vi "Process.vi"(8 "error in":errorcluster, 11 "0MQ_Server":refnum<class "0MQ_Server.lvclass">) -> (0 "error out":errorcluster, 3 "0MQ_Server out":refnum<class "0MQ_Server.lvclass">)   [LabVIEW 2016, in "0MQ_Server.lvclass"]
doc: "---------------------------------------------------------------\nJKI State Machine Objects™\nhttp://jki.net/state-machine-objects/\nCopyright (C) 2005-2015, JKI <info@jki.net>\nALL RIGHTS RESERVED"
uses:
  0MQ_Server.lvclass
  C:/Program Files (x86)/National Instruments/LabVIEW 2016/vi.lib/JKI/JKI SMO/SMO/SMO.lvclass
  <vilib>/JKI/JKI SMO/SMO/Typedefs/Parent Call--Enum.ctl
  <vilib>/addons/zeromq/socket_type.ctl
  <vilib>/addons/zeromq/zmq_socket.lvclass
  <vilib>/addons/zeromq/zmq_context.lvclass
  0MQ_Server.lvclass/0MQ_Server.ctl
  <vilib>/addons/zeromq/socket_options.ctl
  <vilib>/JKI/JKI SMO/SMO/SMO.lvclass
  <vilib>/addons/zeromq/zeromq.lvlib
panel:
  # "For instructions on how to use the JKI State Machine Objects, examples and video tutorials, visit:\nhttp://jki.net/state-machine-objects/\n\nJKI State Machine Objects™\nhttp://jki.net/state-machine-objects/\nCopyright (C) 2005-2015, JKI <info@jki.net>\nALL RIGHTS RESERVED"
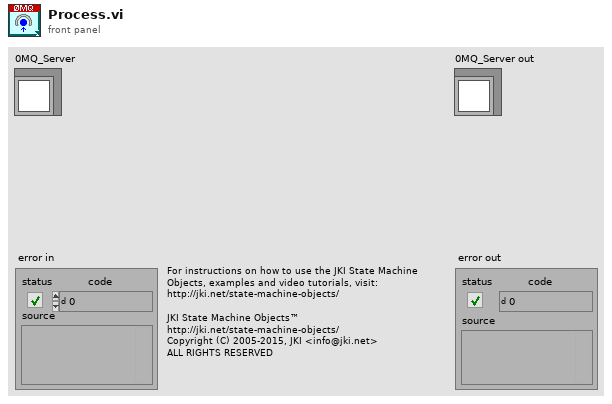
[diagram p1: front panel]
types:
  T1 = typedef "SMO.lvclass/Parent Call--Enum.ctl" = enum16{"Allows parent to run", "Does not request parent to run"}
  T2 = enum32{"invalid app kind", "Development System", "Run Time System", "Student Edition", "Embedded LabVIEW", "Evaluation", "Custom"}
  T3 = enum32{"Invalid", "Standard", "Closed", "Hidden", "Minimized", "Maximized"}
  T4 = enum32{"Bad", "Idle", "Run top level", "Running"}
  T5 = typedef "zeromq.lvlib/socket_options.ctl" = enum8{"NONE", "ZMQ_HWM", "<2>", "ZMQ_SWAP", "ZMQ_AFFINITY", "ZMQ_IDENTITY", "ZMQ_SUBSCRIBE", "ZMQ_UNSUBSCRIBE", "ZMQ_RATE", "ZMQ_RECOVERY_IVL", "ZMQ_MCAST_LOOP", "ZMQ_SNDBUF", "ZMQ_RCVBUF", "ZMQ_RCVMORE", "ZMQ_FD", "ZMQ_EVENTS", "ZMQ_TYPE", "ZMQ_LINGER", "ZMQ_RECONNECT_IVL", "ZMQ_BACKLOG", "ZMQ_RECOVERY_IVL_MSEC", "ZMQ_RECONNECT_IVL_MAX", "ZMQ_MAXMSGSIZE", "ZMQ_SNDHWM", "ZMQ_RCVHWM", "ZMQ_MULTICAST_HOPS", "<26>", "ZMQ_RCVTIMEO", "ZMQ_SNDTIMEO", "<29>", "<30>", "ZMQ_IPV4ONLY", "ZMQ_LAST_ENDPOINT", "ZMQ_ROUTER_MANDATORY", "ZMQ_TCP_KEEPALIVE", "ZMQ_TCP_KEEPALIVE_CNT", "ZMQ_TCP_KEEPALIVE_IDLE", "ZMQ_TCP_KEEPALIVE_INTVL", "ZMQ_TCP_ACCEPT_FILTER", "ZMQ_DELAY_ATTACH_ON_CONNECT", "ZMQ_XPUB_VERBOSE"}
  T6 = typedef "zeromq.lvlib/socket_type.ctl" = enum8{"ZMQ_PAIR", "ZMQ_PUB", "ZMQ_SUB", "ZMQ_REQ", "ZMQ_REP", "ZMQ_DEALER", "ZMQ_ROUTER", "ZMQ_PULL", "ZMQ_PUSH", "ZMQ_XPUB", "ZMQ_XSUB"}
  T7 = typedef "0MQ_Server.lvclass/Socket Config.ctl" = cluster{"Socket type":T6, "endpoint":string, "socket filter":string}
  T8 = cluster{"Core":cluster{"Current VI Reference":refnum<vi>, "Close Panel on Exit?":bool, "error":errorcluster}, "Self Reference":refnum<class "0MQ_Server.lvclass">, "ZMQ Socket":refnum<class "zmq_socket.lvclass">, "ZMQ Context":refnum<class "zmq_context.lvclass">, "Send String":string, "Socket Config":T7, "T_O":i32}
  T9 = cluster{"Current VI Reference":refnum<vi>, "Close Panel on Exit?":bool, "error":errorcluster}
  T10 = typedef "SMO.lvclass/Protected Events.ctl" = cluster{"StopProcesses":refnum<user-event>, "AbortProcesses":refnum<user-event>, "Config Changed":refnum<user-event>, "Dependency":refnum<user-event>}
  T11 = typedef "0MQ_Server.lvclass/0MQ_Server.ProtectedEvents.ctl" = cluster{"SendMessage":refnum<user-event>}
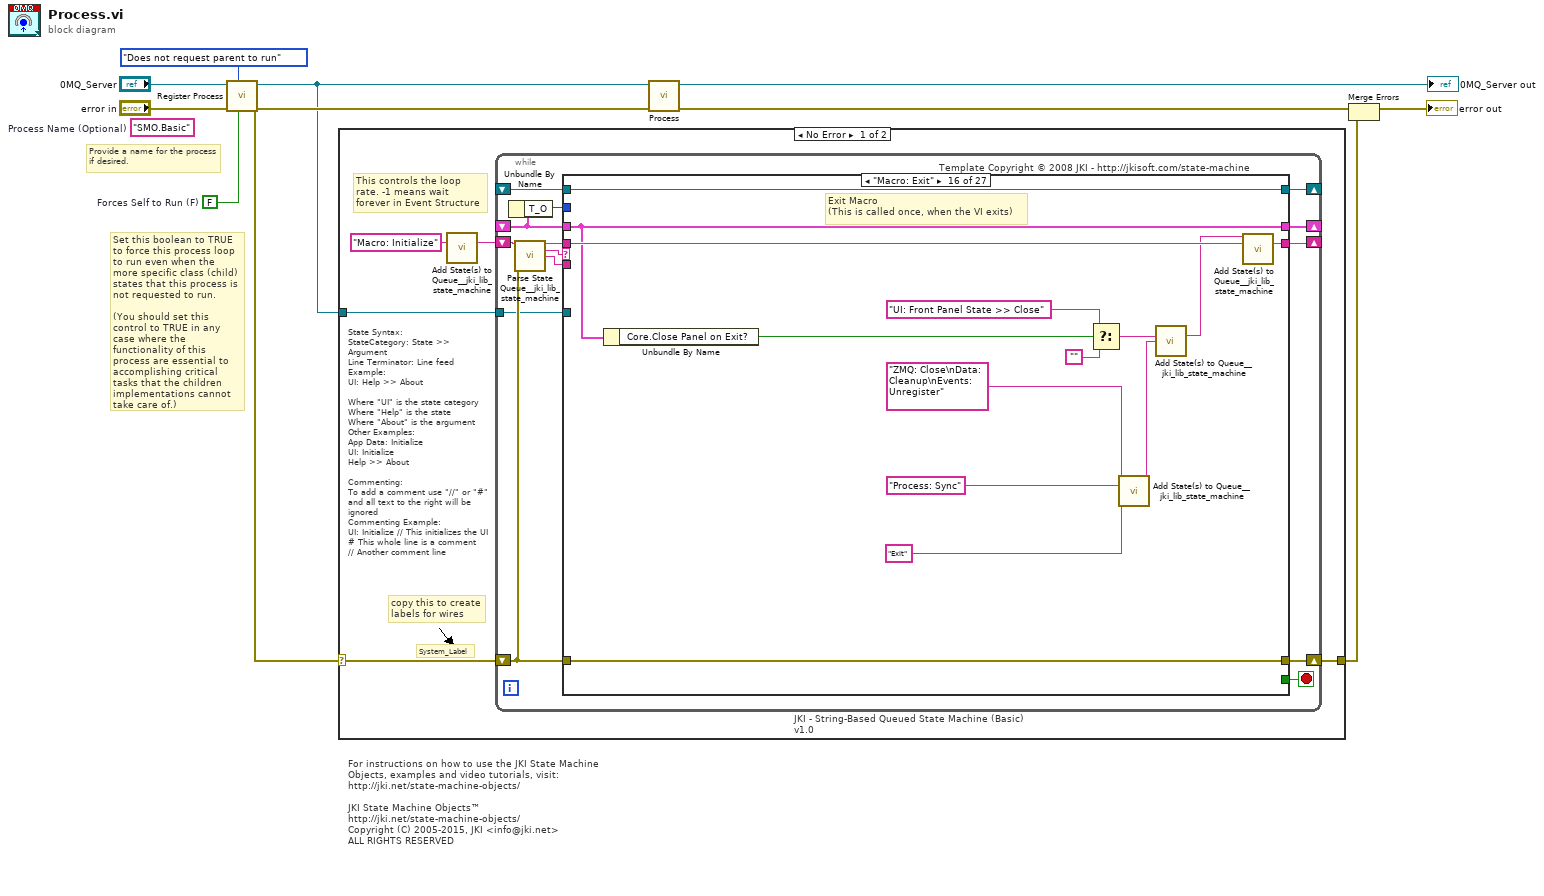
[diagram p0: block diagram]
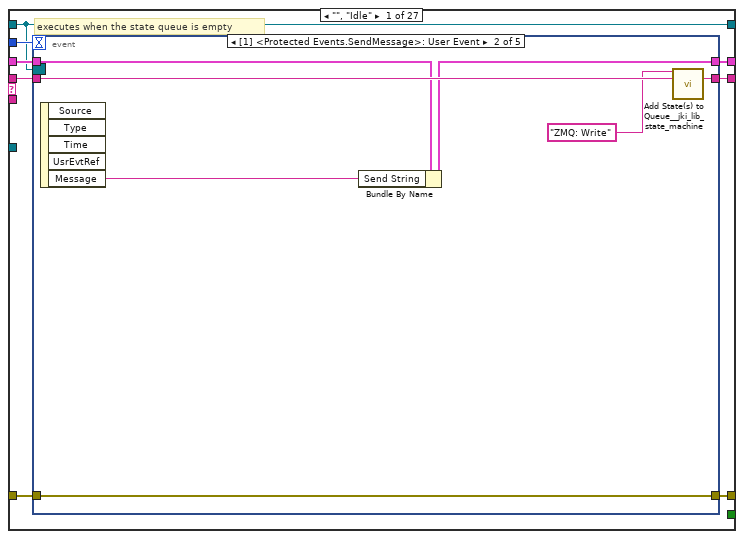
[diagram p2: hidden frame]
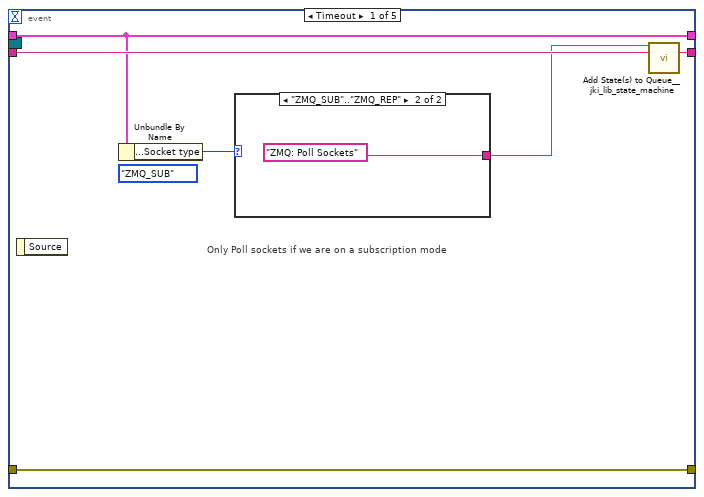
[diagram p3: hidden frame]
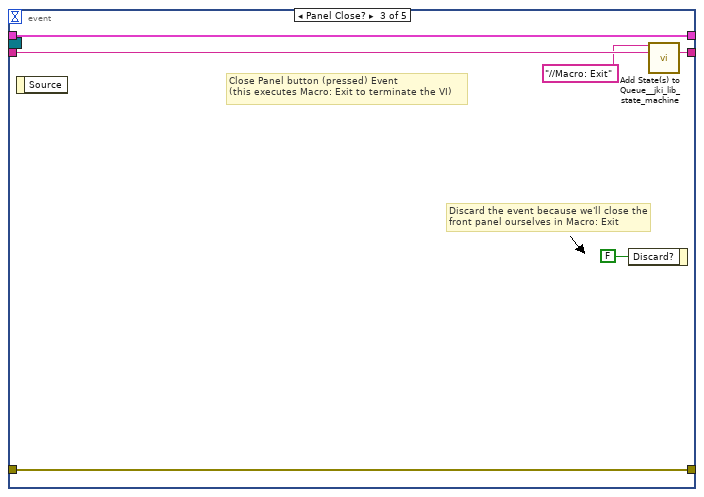
[diagram p5: hidden frame]
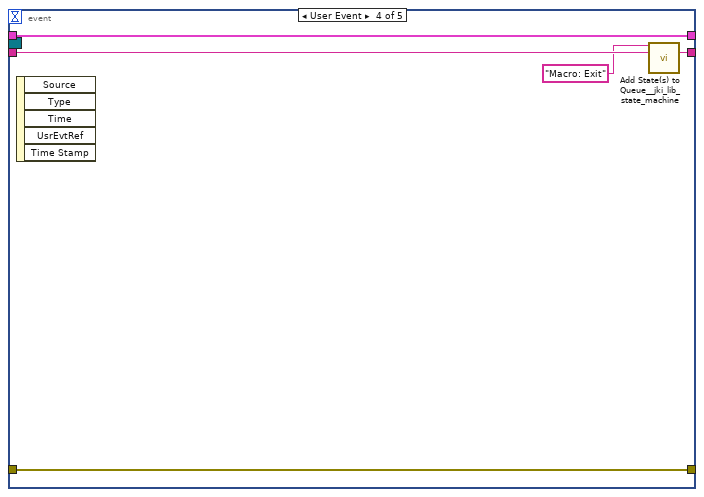
[diagram p6: hidden frame]
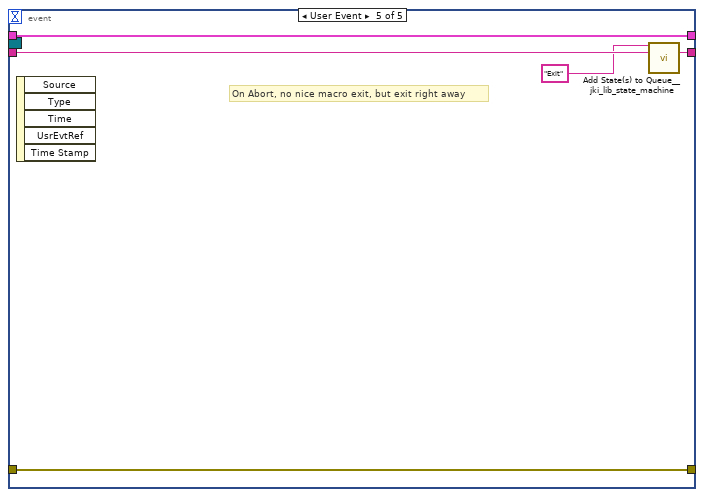
[diagram p7: hidden frame]
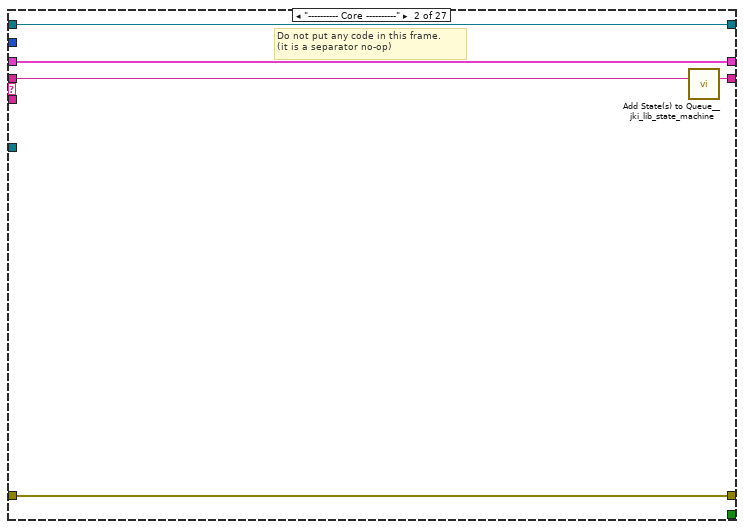
[diagram p8: hidden frame]
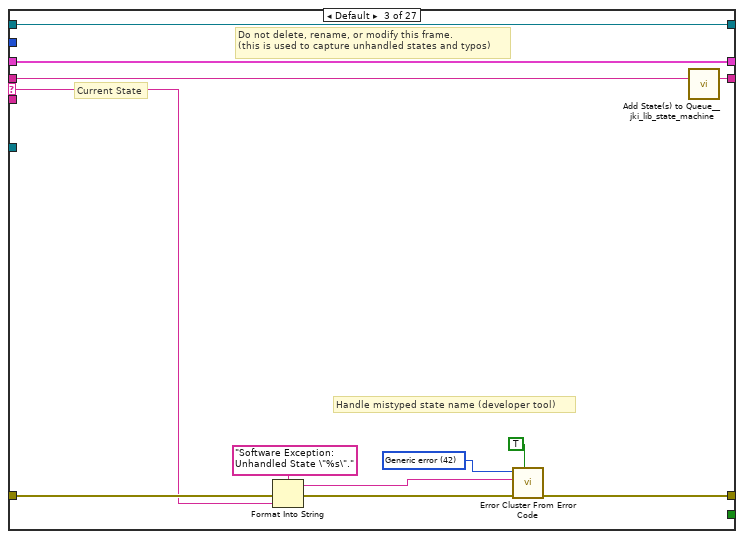
[diagram p9: hidden frame]
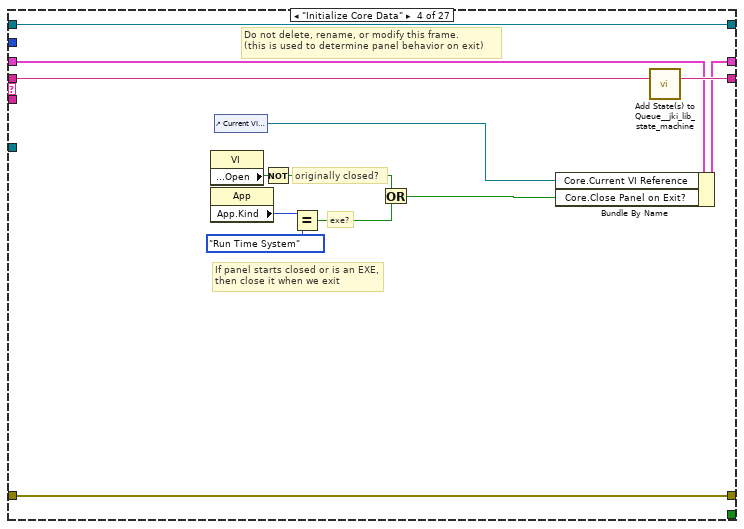
[diagram p10: hidden frame]
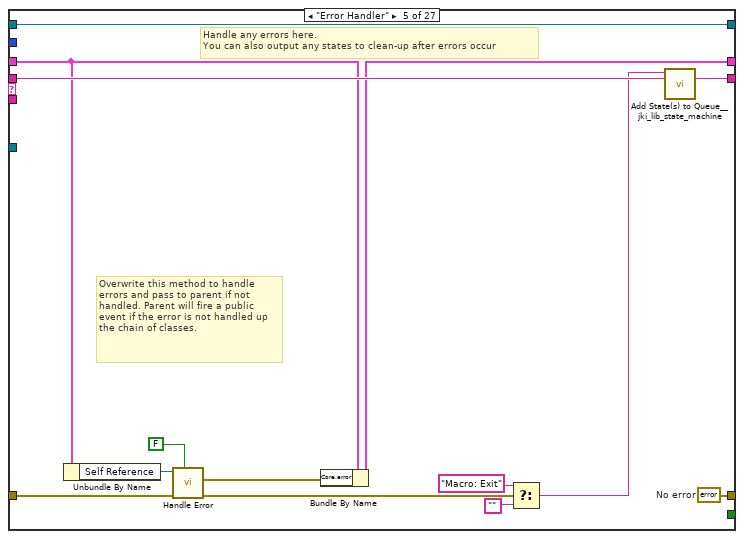
[diagram p11: hidden frame]
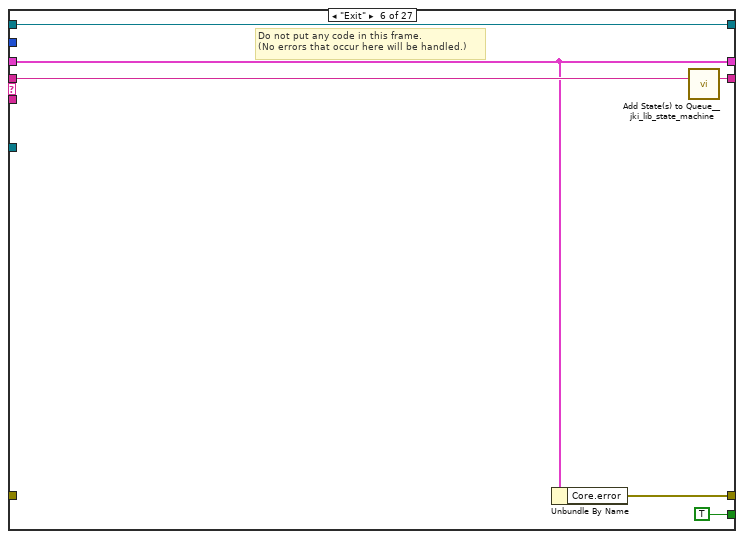
[diagram p12: hidden frame]
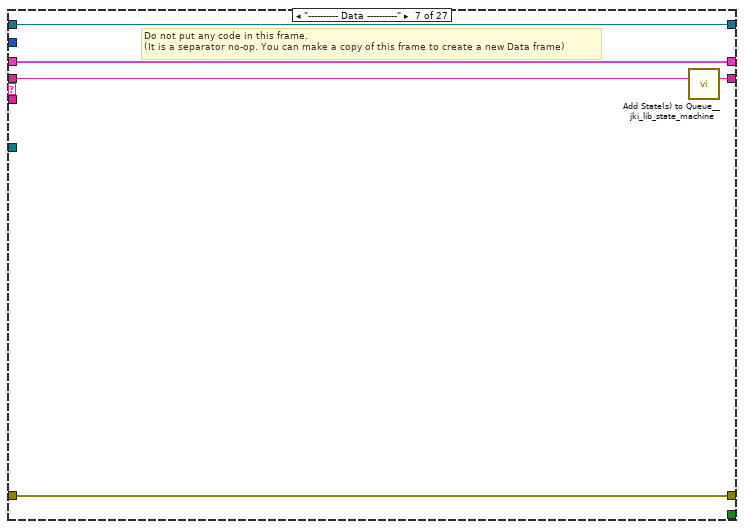
[diagram p13: hidden frame]
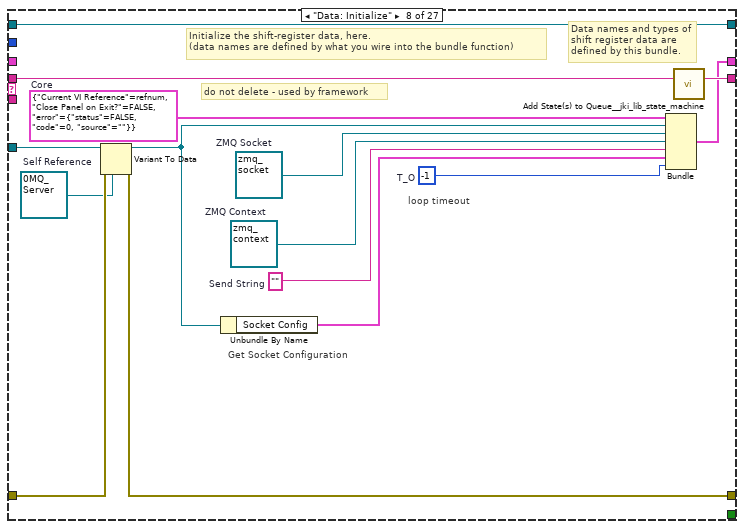
[diagram p14: hidden frame]
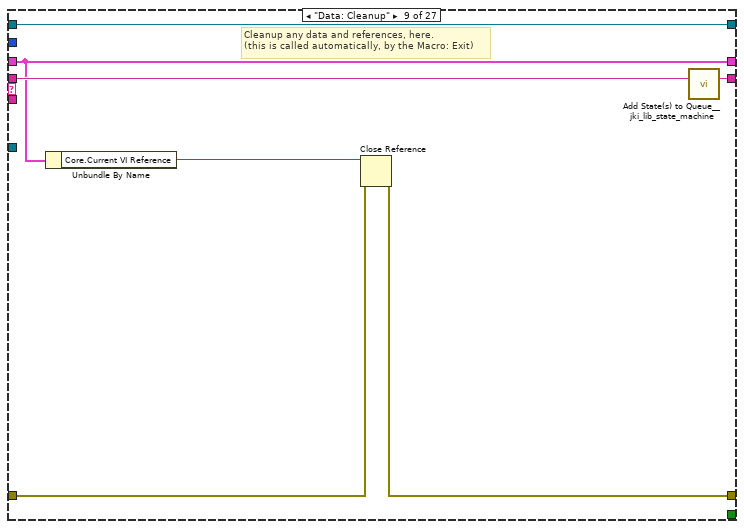
[diagram p15: hidden frame]
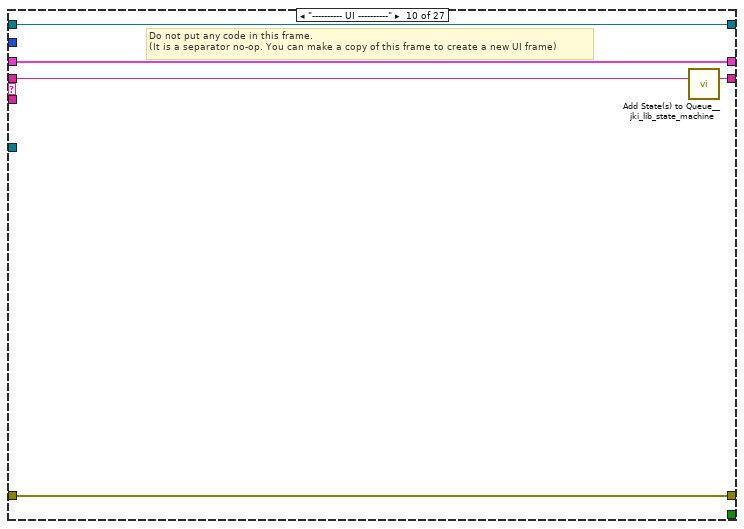
[diagram p16: hidden frame]
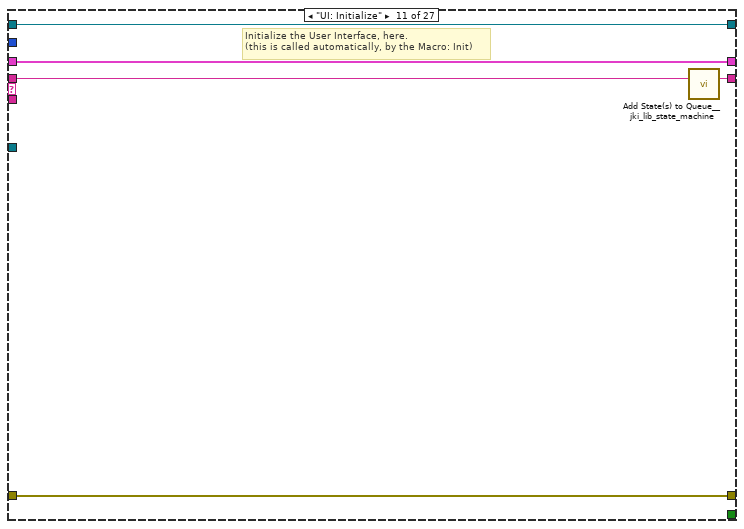
[diagram p17: hidden frame]
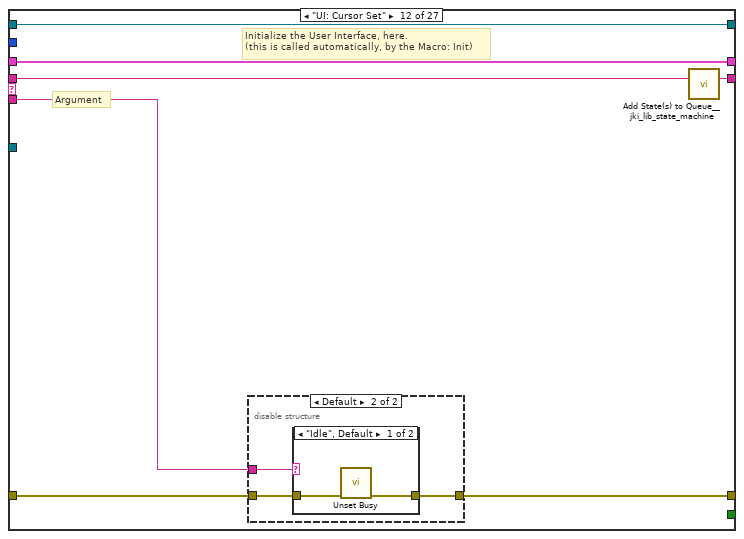
[diagram p18: hidden frame]
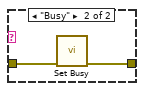
[diagram p20: hidden frame]
diagram:
  w1 = FALSE  # Forces Self to Run (F)
  (unwired) "SMO.Basic"  # Process Name (Optional)
  # "Provide a name for the process\nif desired."
  # "Set this boolean to TRUE to force this process loop to run even when the more specific class (child) states that this process is not requested to run.\n\n(You should set this control to TRUE in any case where the functionality of this process are essential to accomplishing critical tasks that the children implementations cannot take care of.)"
  # "For instructions on how to use the JKI State Machine Objects, examples and video tutorials, visit:\nhttp://jki.net/state-machine-objects/\n\nJKI State Machine Objects™\nhttp://jki.net/state-machine-objects/\nCopyright (C) 2005-2015, JKI <info@jki.net>\nALL RIGHTS RESERVED"
  n1 = call <vilib>:"Register Process.vi"("Forces Self to Run (F)"=w1, "Parent Call"=Parent_Call--Enum."Does not request parent to run", "error in (no error)"="error in", "SMO"="0MQ_Server") -> ("error out"=w7:errorcluster, "SMO out"=w6:refnum<class "0MQ_Server.lvclass">)  [unwired: 6 in]
  n2 = case shown="No Error" w7 {
    selector: w7 -> [w12 w391]
    tunnel: w6 -> [w13 _]
    tunnel: [w11 w391] -> w3
    frame No Error {
      # "State Syntax:\nStateCategory: State >> Argument\nLine Terminator: Line feed\nExample:\nUI: Help >> About\n\nWhere \"UI\" is the state category\nWhere \"Help\" is the state\nWhere \"About\" is the argument\nOther Examples:\nApp Data: Initialize\nUI: Initialize\nHelp >> About\n\nCommenting:\nTo add a comment use \"//\" or \"#\" and all text to the right will be ignored\nCommenting Example:\nUI: Initialize // This initializes the UI\n# This whole line is a comment\n// Another comment line"
      # "copy this to create labels for wires"
      # "This controls the loop rate. -1 means wait forever in Event Structure"
      # "System_Label"
      n3 = call <vilib>:"Add State(s) to Queue__jki_lib_state_machine.vi"("State(s) in (\"\")"="Macro: Initialize") -> ("States Out"=w15:string)  [unwired: 14 in]
      n4 = while "JKI - String-Based Queued State Machine (Basic) v1.0" {
        shift-right: [w22] -> _
        shift-left: _ -> [w17]
        shift-right: [w25] -> w11
        shift-left: w12 -> [w21]
        shift-right: [w24] -> _
        shift-left: w15 -> [w26]
        tunnel: w13 -> [w20]
        shift-right: [w19] -> _
        shift-left: _ -> [w18]
        stop <- w23 stop-if-true
        # "Template Copyright © 2008 JKI - http://jkisoft.com/state-machine"
        n5 = Unbundle By Name(w17) -> ("T_O"=w16:i32)
        n6 = call <vilib>:"Parse State Queue__jki_lib_state_machine.vi"("State Queue"=w26, "Error In (no error)"=w21) -> ("Remaining States"=w28:string, "Current State"=w29:string, "Arguments"=w27:string)  [unwired: 11 in]
        n7 = case shown="\"Macro: Exit\"" w29 {
          selector: w29 -> [_ _ w74 _ _ _ _ _ _ _ _ _ _ _ _ _ _ _ _ _ _ _ _ _ _ _ _]
          tunnel: w28 -> [w37 w72 w78 w97 w111 w117 w122 w137 w144 w149 w154 w161 w177 w209 w223 w237 w242 w253 w258 w272 w288 w293 w305 w318 w358 w367 w384]
          tunnel: w27 -> [_ _ _ _ _ _ _ _ _ _ _ w155 w171 _ _ _ _ _ _ _ _ _ _ _ _ _ _]
          tunnel: w17 -> [w35 w69 w76 w88 w100 w113 w119 _ w139 w146 w152 w159 w173 w206 w219 w228 w239 w250 w255 w270 w286 w291 w294 w314 w354 w364 w381]
          tunnel: [w34 w70 w80 w94 w102 w112 w120 w133 w140 w147 w151 w156 w174 w207 w221 w235 w240 w244 w256 w268 w283 w289 w296 w309 w351 w361 w379] -> w25
          tunnel: w21 -> [w33 w70 w79 w94 w107 _ w120 w134 w141 w147 w151 w157 w175 w207 w221 w235 w240 w245 w256 w269 w284 w289 w297 w310 w352 w362 w380]
          tunnel: [w36 w71 w77 w96 w110 w116 w121 w136 w143 w148 w153 w160 w176 w208 w222 w236 w241 w252 w257 w271 w287 w292 w304 w317 w357 w366 w383] -> w24
          tunnel: [_ _ _ _ _ TRUE _ _ _ _ _ _ _ _ _ _ _ _ _ _ _ _ _ _ _ _ _] -> w23
          tunnel: [w32 w69 w76 w95 w99 w113 w119 w135 w139 w146 w152 w159 w173 w206 w219 w228 w239 w250 w255 w270 w286 w291 w300 w315 w354 w364 w381] -> w22
          tunnel: w16 -> [w31 _ _ _ _ _ _ _ _ _ _ _ _ _ _ _ _ _ _ _ _ _ _ _ _ _ _]
          tunnel: w20 -> [_ _ _ _ _ _ _ w131 _ _ _ _ _ _ _ _ _ _ _ _ _ _ _ _ _ _ _]
          tunnel: [w30 w68 w73 w85 w109 w114 w118 w130 w138 w145 w150 w158 w170 w205 w220 w229 w238 w251 w254 w267 w285 w290 w303 w316 w356 w365 w382] -> w19
          tunnel: w18 -> [w30 w68 w73 w85 w109 w114 w118 w130 w138 w145 w150 w158 w170 w205 w220 w229 w238 w251 w254 w263 w285 w290 w303 w316 w356 w365 w382]
          frame "", "Idle" {
            # "executes when the state queue is empty"
            n8 = event shown="[1] <Protected Events.SendMessage>: User Event" {
              selector: w30 -> [_ _ _ _ _]
              dyn-events: _ -> [_ _ _ _ _]
              timeout: w31 -> [_ _ _ _ _]
              tunnel: w37 -> [w43 w51 w57 w62 w67]
              tunnel: [w42 w50 w56 w61 w66] -> w36
              tunnel: w35 -> [w40 w48 w54 w59 w64]
              tunnel: [w41 w49 w55 w60 w65] -> w34
              tunnel: w33 -> [w41 w49 w55 w60 w65]
              tunnel: [w40 w47 w54 w59 w64] -> w32
              event Timeout {
                (unwired) socket_type."ZMQ_SUB" ("y")
                # "Only Poll sockets if we are on a subscription mode"
                n9 = event-data() -> ()  [unwired: 1 in, 1 out]
                n10 = Unbundle By Name(w40) -> ("Socket Config.Socket type"=w38:T6)
                n11 = case shown="\"ZMQ_SUB\"..\"ZMQ_REP\"" w38 {
                  tunnel: [_ "ZMQ: Poll Sockets" ("State(s) in Front (\"\")")] -> w39
                  frame Default {
                  }
                  frame "ZMQ_SUB".."ZMQ_REP" {
                  }
                }
                n12 = call <vilib>:"Add State(s) to Queue__jki_lib_state_machine.vi"("State(s) in Front (\"\")"=w39, "State(s) in (\"\")"=w43) -> ("States Out"=w42:string)  [unwired: 13 in]
              }
              event User Event {
                n13 = event-data() -> ("Message"=w46:string)  [unwired: 1 in, 4 out]
                n14 = Bundle By Name(cluster=w48, "Send String"=w46) -> (w47:T8)
                n15 = call <vilib>:"Add State(s) to Queue__jki_lib_state_machine.vi"("State(s) in Front (\"\")"="ZMQ: Write" ("State(s) in Front (\"\")"), "State(s) in (\"\")"=w51) -> ("States Out"=w50:string)  [unwired: 13 in]
              }
              event Panel Close? {
                # "Discard the event because we'll close the front panel ourselves in Macro: Exit"
                # "Close Panel button (pressed) Event\n(this executes Macro: Exit to terminate the VI)"
                n16 = event-data() -> ()  [unwired: 1 in, 1 out]
                n17 = event-data("Discard?"=FALSE) -> ()  [unwired: 1 in, 1 out]
                n18 = call <vilib>:"Add State(s) to Queue__jki_lib_state_machine.vi"("State(s) in Front (\"\")"="//Macro: Exit", "State(s) in (\"\")"=w57) -> ("States Out"=w56:string)  [unwired: 13 in]
              }
              event User Event {
                n19 = event-data() -> ()  [unwired: 1 in, 5 out]
                n20 = call <vilib>:"Add State(s) to Queue__jki_lib_state_machine.vi"("State(s) in Front (\"\")"="Macro: Exit", "State(s) in (\"\")"=w62) -> ("States Out"=w61:string)  [unwired: 13 in]
              }
              event User Event {
                # "On Abort, no nice macro exit, but exit right away"
                n21 = event-data() -> ()  [unwired: 1 in, 5 out]
                n22 = call <vilib>:"Add State(s) to Queue__jki_lib_state_machine.vi"("State(s) in Front (\"\")"="Exit", "State(s) in (\"\")"=w67) -> ("States Out"=w66:string)  [unwired: 13 in]
              }
            }
          }
          frame "---------- Core ----------" {
            # "Do not put any code in this frame.\n(it is a separator no-op)"
            n23 = call <vilib>:"Add State(s) to Queue__jki_lib_state_machine.vi"("State(s) in (\"\")"=w72) -> ("States Out"=w71:string)  [unwired: 14 in]
          }
          frame Default {
            w83 = 42 items=["No error", "Argument error", "Memory is full", "Out of zone", "End of file", "File already open", "Generic file I/O error", "File not found", "File permission error", "Disk is full", "Duplicate path", "Too many files open", "System feature not enabled", "Resource file not found", "Cannot add resource", "Resource not found", "Image not found", "Image memory error", "Pen does not exist", "Config type invalid", "Config token not found", "Config parse error", "Config memory error", "Bad external code format", "Bad external code offset", "External code not present", "Null window", "Destroy window error", "Null menu", "Print aborted", "Bad print record", "Print driver error", "Windows error during printing", "Memory error during printing", "Print dialog error", "Generic print error", "Invalid device refnum", "Device not found", "Device parameter error", "Device unit error", "Cannot open device", "Device call aborted", "Generic error", "Cancelled by user", "Object ID too low", "Object ID too high", "Object not in heap", "Unknown heap", "Unknown object (invalid DefProc)", "Unknown object (DefProc not in table)", "Message out of range", "Invalid (null) method", "Unknown message", "Manager call not supported", "Bad address", "Network operation in progress", "Network operation timed out", "Connection is busy", "Network attribute not supported", "Network error", "Address in use", "System out of memory", "Connection aborted", "Connection refused", "Not connected", "Already connected", "Connection closed", "Initialization error (interapplication manager)", "Bad occurrence", "Wait on unbound occurrence handler", "Occurrence queue overflow", "Datalog type conflict", "Unused", "Unrecognized type (interapplication manager)", "Memory corrupt", "Failed to make temporary DLL", "Old CIN version", "Drag socket not found", "Failed to load drop-object", "Failed to register OLE object", "Failed to release OLE object", "Format specifier type mismatch", "Unknown format specifier", "Too few format specifiers", "Too many format specifiers", "Scan failed", "Newer CIN version", "Error converting to variant", "Runtime menu error", "Password tampered", "Variant attribute not found", "Incompatible variant data type", "Event data is not available", "Event Store is not present", "Occurrence is not found", "Event Queue is not created", "Event info is not available", "Refnum passed is NULL", "Error retrieving Class GUID", "Error retrieving CoClass GUID", "Error retrieving TypeLib GUID.", "Bad built application magic bytes.", "Specific driver is different from the specific driver associated with the Logical Name.", "There is no session opened to the class driver.", "Max Error", "MAX - Error with config objects", "MAX - Error loading configuration", "MAX - Group not supported"]
            # "Current State"
            # "Do not delete, rename, or modify this frame.\n(this is used to capture unhandled states and typos)"
            # "Handle mistyped state name (developer tool)"
            n24 = Format Into String(format string="Software Exception: Unhandled State \"%s\"." ("message"), error in=w79, w74) -> (resulting string=w82:string, error out=w81:errorcluster)  [unwired: 1 in]
            n25 = call <vilib>:"Error Cluster From Error Code.vi"("show call chain? (False)"=TRUE, "error in (no error)"=w81, "error message (\"\")"=w82, "error code (0)"=w83) -> ("error out"=w80:errorcluster)  [unwired: 5 in]
            n26 = call <vilib>:"Add State(s) to Queue__jki_lib_state_machine.vi"("State(s) in (\"\")"=w78) -> ("States Out"=w77:string)  [unwired: 14 in]
          }
          frame "Initialize Core Data" {
            # "Do not delete, rename, or modify this frame.\n(this is used to determine panel behavior on exit)"
            # "originally closed?"
            # "exe?"
            # "If panel starts closed or is an EXE, then close it when we exit"
            n27 = property class="VI"() -> ("Front Panel.Open"=w93:bool)  [unwired: 2 in, 2 out]
            n28 = property class="App"() -> ("App.Kind"=w92:T2)  [unwired: 2 in, 2 out]
            n29 = control-ref of="Current VI Reference"() -> (w86:refnum<vi>)
            n30 = Not(x=w93) -> (.not. x?=w90:bool)
            n31 = Equal?(x=w92, y=T2."Run Time System" ("Application:Kind")) -> (x = y?=w89:bool)
            n32 = Or(x=w90, y=w89) -> (x .or. y?=w87:bool)
            n33 = Bundle By Name(cluster=w88, "Core.Current VI Reference"=w86, "Core.Close Panel on Exit?"=w87) -> (w95:T8)
            n34 = call <vilib>:"Add State(s) to Queue__jki_lib_state_machine.vi"("State(s) in (\"\")"=w97) -> ("States Out"=w96:string)  [unwired: 14 in]
          }
          frame "Error Handler" {
            w102 = errorcluster {"status"=FALSE, "code"=0, "source"=""}  # No error
            # "Overwrite this method to handle errors and pass to parent if not handled. Parent will fire a public event if the error is not handled up the chain of classes."
            # "Handle any errors here.\nYou can also output any states to clean-up after errors occur"
            n35 = Unbundle By Name(w100) -> ("Self Reference"=w108:refnum<class "0MQ_Server.lvclass">)
            n36 = call-dynamic "Handle Error.vi"("Stop on Unhandled Error (T)"=FALSE, "error in"=w107, "SMO"=w108) -> ("handling error"=w103:errorcluster, "Unhandled error"=w101:errorcluster)  [unwired: 6 in, 1 out]
            n37 = Bundle By Name(cluster=w100, "Core.error"=w101) -> (w99:T8)
            n38 = Select(t="Macro: Exit", s=w103, f="") -> (s? t:f=w104:string)
            n39 = call <vilib>:"Add State(s) to Queue__jki_lib_state_machine.vi"("State(s) in Front (\"\")"=w104, "State(s) in (\"\")"=w111) -> ("States Out"=w110:string)  [unwired: 13 in]
          }
          frame "Exit" {
            # "Do not put any code in this frame.\n(No errors that occur here will be handled.)"
            n40 = Unbundle By Name(w113) -> ("Core.error"=w112:errorcluster)
            n41 = call <vilib>:"Add State(s) to Queue__jki_lib_state_machine.vi"("State(s) in (\"\")"=w117) -> ("States Out"=w116:string)  [unwired: 14 in]
          }
          frame "---------- Data ----------" {
            # "Do not put any code in this frame.\n(It is a separator no-op. You can make a copy of this frame to create a new Data frame)"
            n42 = call <vilib>:"Add State(s) to Queue__jki_lib_state_machine.vi"("State(s) in (\"\")"=w122) -> ("States Out"=w121:string)  [unwired: 14 in]
          }
          frame "Data: Initialize" {
            w123 = -1  # T_O
            w126 = ""  # Send String
            w127 = refnum<class "zmq_context.lvclass"> refnum  # ZMQ Context
            w128 = refnum<class "zmq_socket.lvclass"> refnum  # ZMQ Socket
            w129 = T9 {"Current VI Reference"=refnum, "Close Panel on Exit?"=FALSE, "error"={"status"=FALSE, "code"=0, "source"=""}}  # Core
            w132 = refnum<class "0MQ_Server.lvclass"> refnum  # Self Reference
            # "loop timeout"
            # "Get Socket Configuration"
            # "do not delete - used by framework"
            # "Data names and types of shift register data are defined by this bundle."
            # "Initialize the shift-register data, here.\n(data names are defined by what you wire into the bundle function)"
            n43 = Variant To Data(error in=w134, type=w132, Variant=w131) -> (data=w125:refnum<class "0MQ_Server.lvclass">, error out=w133:errorcluster)
            n44 = Unbundle By Name(w125) -> ("Socket Config"=w124:T7)
            n45 = Bundle("Core"=w129, "Self Reference"=w125, "ZMQ Socket"=w128, "ZMQ Context"=w127, "Send String"=w126, "Socket Config"=w124, "T_O"=w123) -> (w135:T8)  [unwired: 1 in]
            n46 = call <vilib>:"Add State(s) to Queue__jki_lib_state_machine.vi"("State(s) in (\"\")"=w137) -> ("States Out"=w136:string)  [unwired: 14 in]
          }
          frame "Data: Cleanup" {
            # "Cleanup any data and references, here.\n(this is called automatically, by the Macro: Exit)"
            n47 = Unbundle By Name(w139) -> ("Core.Current VI Reference"=w142:refnum<vi>)
            n48 = Close Reference(reference=w142, error in (no error)=w141) -> (error out=w140:errorcluster)
            n49 = call <vilib>:"Add State(s) to Queue__jki_lib_state_machine.vi"("State(s) in (\"\")"=w144) -> ("States Out"=w143:string)  [unwired: 14 in]
          }
          frame "---------- UI ----------" {
            # "Do not put any code in this frame.\n(It is a separator no-op. You can make a copy of this frame to create a new UI frame)"
            n50 = call <vilib>:"Add State(s) to Queue__jki_lib_state_machine.vi"("State(s) in (\"\")"=w149) -> ("States Out"=w148:string)  [unwired: 14 in]
          }
          frame "UI: Initialize" {
            # "Initialize the User Interface, here.\n(this is called automatically, by the Macro: Init)"
            n51 = call <vilib>:"Add State(s) to Queue__jki_lib_state_machine.vi"("State(s) in (\"\")"=w154) -> ("States Out"=w153:string)  [unwired: 14 in]
          }
          frame "UI: Cursor Set" {
            # "Argument"
            # "Initialize the User Interface, here.\n(this is called automatically, by the Macro: Init)"
            n52 = disable-structure shown="Default" {
              disable-tunnel: w157 -> [w162 w165]
              disable-tunnel: [w162 w164] -> w156
              disable-tunnel: w155 -> [_ w163]
              frame condition #0 {
              }
              frame condition #1 (active) {
                n53 = case shown="\"Idle\", Default" w163 {
                  tunnel: w165 -> [w167 w169]
                  tunnel: [w166 w168] -> w164
                  frame "Idle", Default {
                    n54 = call <vilib>:"Unset Busy.vi"("error in (no error)"=w167) -> ("error out"=w166:errorcluster)  [unwired: 10 in]
                  }
                  frame "Busy" {
                    n55 = call <vilib>:"Set Busy.vi"("error in (no error)"=w169) -> ("error out"=w168:errorcluster)  [unwired: 9 in, 1 out]
                  }
                }
              }
            }
            n56 = call <vilib>:"Add State(s) to Queue__jki_lib_state_machine.vi"("State(s) in (\"\")"=w161) -> ("States Out"=w160:string)  [unwired: 14 in]
          }
          frame "UI: Front Panel State" {
            # "Argument"
            # "Set Front Panel Open or Closed\n(Usage: \"UI: Front Panel State >> Open|Close\")"
            n57 = Unbundle By Name(w173) -> ("Core.Current VI Reference"=w172:refnum<vi>)
            n58 = disable-structure shown="Default" {
              disable-tunnel: w175 -> [w181 w204]
              disable-tunnel: [w180 w204] -> w174
              disable-tunnel: w172 -> [w179 _]
              disable-tunnel: w171 -> [w178 _]
              frame condition #0 (active) {
                n59 = case shown="\"Close\"" w178 {
                  tunnel: w181 -> [w185 w198]
                  tunnel: [w187 w199] -> w180
                  tunnel: w179 -> [w186 w196]
                  frame "Open", Default {
                    n60 = property class="VI"(reference=w186, error in=w185) -> (reference out=w183:refnum<vi>, error out=w184:errorcluster, "FP.State"=w182:T3)
                    n61 = case shown="\"Closed\"" w182 {
                      tunnel: [w190 w193] -> w187
                      tunnel: w184 -> [w189 w193]
                      tunnel: w183 -> [w188 _]
                      frame "Closed" {
                        n62 = invoke class="VI" method="FP.Open"(reference=w188, error in=w189, "Activate"=TRUE, "State"=T3."Standard") -> (error out=w190:errorcluster)  [unwired: 1 in, 4 out]
                      }
                      frame Default {
                      }
                    }
                  }
                  frame "Close" {
                    n63 = property class="VI"(reference=w196, error in=w198) -> (reference out=w195:refnum<vi>, error out=w197:errorcluster, "FP.State"=w194:T3)
                    n64 = case shown="Default" w194 {
                      tunnel: [w200 w203] -> w199
                      tunnel: w197 -> [w200 w202]
                      tunnel: w195 -> [_ w201]
                      frame "Invalid", "Closed" {
                      }
                      frame Default {
                        n65 = invoke class="VI" method="FP.Close"(reference=w201, error in=w202) -> (error out=w203:errorcluster)  [unwired: 1 in, 2 out]
                      }
                    }
                  }
                }
              }
              frame condition #1 {
              }
            }
            n66 = call <vilib>:"Add State(s) to Queue__jki_lib_state_machine.vi"("State(s) in (\"\")"=w177) -> ("States Out"=w176:string)  [unwired: 14 in]
          }
          frame "---------- Macro ----------" {
            # "Do not put any code in this frame.\n(It is a separator no-op. You can make a copy of this frame to create a new Macro frame)"
            n67 = call <vilib>:"Add State(s) to Queue__jki_lib_state_machine.vi"("State(s) in (\"\")"=w209) -> ("States Out"=w208:string)  [unwired: 14 in]
          }
          frame "Macro: Initialize" {
            w214 = "UI: Initialize\nUI: Front Panel State >> Open\nZMQ: Initialize\nZMQ: Create Socket"  # UI: Initialize UI: Front Panel State >> Open ZMQ: Initialize ZMQ: Create Socket
            w210 = "Process: Sync"
            # "Initialization Macro\n(This is called once, when the VI starts)"
            n68 = control-ref of="This VI"() -> (w212:refnum<vi>)
            n69 = property class="VI"(reference=w212) -> ("Exec.State"=w211:T4)  [unwired: 1 in, 2 out]
            n70 = Equal?(x=w211, y=T4."Run top level") -> (x = y?=w217:bool)
            n71 = Select(t=w210, s=w217, f="") -> ()  [unwired: 1 out]
            n72 = call <vilib>:"Add State(s) to Queue__jki_lib_state_machine.vi"("State(s) in Front (\"\")"="Data: Initialize\nInitialize Core Data\nEvents: Register", "State(s) in (\"\")"=w210, "State(s) at Back (\"\")"=w214) -> ("States Out"=w213:string)  [unwired: 12 in]
            n73 = call <vilib>:"Add State(s) to Queue__jki_lib_state_machine.vi"("State(s) in Front (\"\")"=w213, "State(s) in (\"\")"=w223) -> ("States Out"=w222:string)  [unwired: 13 in]
          }
          frame "Macro: Exit" {
            # "Exit Macro\n(This is called once, when the VI exits)"
            n74 = Unbundle By Name(w228) -> ("Core.Close Panel on Exit?"=w234:bool)
            n75 = Select(t="UI: Front Panel State >> Close", s=w234, f="") -> (s? t:f=w231:string)
            n76 = call <vilib>:"Add State(s) to Queue__jki_lib_state_machine.vi"("State(s) in Front (\"\")"="ZMQ: Close\nData: Cleanup\nEvents: Unregister", "State(s) in (\"\")"="Process: Sync", "State(s) at Back (\"\")"="Exit") -> ("States Out"=w225:string)  [unwired: 12 in]
            n77 = call <vilib>:"Add State(s) to Queue__jki_lib_state_machine.vi"("State(s) in (\"\")"=w231, "State(s) at Back (\"\")"=w225) -> ("States Out"=w230:string)  [unwired: 13 in]
            n78 = call <vilib>:"Add State(s) to Queue__jki_lib_state_machine.vi"("State(s) in Front (\"\")"=w230, "State(s) in (\"\")"=w237) -> ("States Out"=w236:string)  [unwired: 13 in]
          }
          frame "---------- Process ----------" {
            # "Template Separator\n(You can make a copy of, or modify, this frame)"
            n79 = call <vilib>:"Add State(s) to Queue__jki_lib_state_machine.vi"("State(s) in (\"\")"=w242) -> ("States Out"=w241:string)  [unwired: 14 in]
          }
          frame "Process: Sync" {
            n80 = Unbundle By Name(w250) -> ("Self Reference"=w246:refnum<class "0MQ_Server.lvclass">)
            n81 = call <vilib>:"WaitOnProcessSync.vi"("error in (no error)"=w245, "SMO"=w246) -> ("error out"=w244:errorcluster, "Don't run?"=w249:bool)  [unwired: 7 in, 1 out]
            n82 = Select(t="Data: Cleanup\nEvents: Unregister\nExit", s=w249, f="") -> (s? t:f=w243:string)
            n83 = call <vilib>:"Add State(s) to Queue__jki_lib_state_machine.vi"("State(s) in Front (\"\")"=w243, "State(s) in (\"\")"=w253) -> ("States Out"=w252:string)  [unwired: 13 in]
          }
          frame "---------- Events ----------" {
            # "Template Separator\n(You can make a copy of, or modify, this frame)"
            n84 = call <vilib>:"Add State(s) to Queue__jki_lib_state_machine.vi"("State(s) in (\"\")"=w258) -> ("States Out"=w257:string)  [unwired: 14 in]
          }
          frame "Events: Register" {
            # "Base Class Protected Events"
            n85 = Unbundle By Name(w270) -> ("Self Reference"=w265:refnum<class "0MQ_Server.lvclass">)
            n86 = call <vilib>:"GetProtectedEvents.vi"("error in (no error)"=w269, "SMO"=w265) -> ("error out"=w261:errorcluster, "SMO Protected Events"=w266:T10, "SMO out"=w262:refnum<class "0MQ_Server.lvclass">)  [unwired: 7 in]
            n87 = call "Read Protected Event.vi"("error in (no error)"=w261, "0MQ_Server in"=w262) -> ("error out"=w260:errorcluster, "Protected Events"=w259:T11)  [unwired: 7 in, 1 out]
            n88 = Not A Number/Path/Refnum?(number/path/refnum=w263) -> (NaN/Path/Refnum?=w264:bool)
            n89 = case shown="True" w264 {
              tunnel: [w277 w282] -> w268
              tunnel: [w276 w281] -> w267
              tunnel: w266 -> [w275 w280]
              tunnel: w260 -> [w274 w279]
              tunnel: w263 -> [_ w278]
              tunnel: w259 -> [w273 _]
              frame True {
                # "Expand to add\nmore events"
                n90 = register-events(error in=w274, w275, w273) -> (reference out=w276:refnum<event-registration>, error out=w277:errorcluster)  [unwired: 1 in]
              }
              frame False {
                n91 = register-events(reference=w278, error in=w279, w280) -> (reference out=w281:refnum<event-registration>, error out=w282:errorcluster)  [unwired: 1 in]
              }
            }
            n92 = call <vilib>:"Add State(s) to Queue__jki_lib_state_machine.vi"("State(s) in (\"\")"=w272) -> ("States Out"=w271:string)  [unwired: 14 in]
          }
          frame "Events: Unregister" {
            n93 = Unregister For Events(event registration refnum=w285, error in=w284) -> (error out=w283:errorcluster)
            n94 = call <vilib>:"Add State(s) to Queue__jki_lib_state_machine.vi"("State(s) in (\"\")"=w288) -> ("States Out"=w287:string)  [unwired: 14 in]
          }
          frame "---------- ZMQ----------" {
            n95 = call <vilib>:"Add State(s) to Queue__jki_lib_state_machine.vi"("State(s) in (\"\")"=w293) -> ("States Out"=w292:string)  [unwired: 14 in]
          }
          frame "ZMQ: Initialize" {
            # "These are common for any ZMQ type"
            # "create socket"
            # "create context"
            n96 = Unbundle By Name(w294) -> ("Socket Config.Socket type"=w298:T6)
            n97 = call <vilib>:"zmq_ctx_create.vi"("error in"=w297) -> ("error out"=w301:errorcluster, "context out"=w302:refnum<class "zmq_context.lvclass">)  [unwired: 3 in]
            n98 = call <vilib>:"zmq_socket.vi"("error in"=w301, "socket type"=w298, "context in"=w302) -> ("error out"=w296:errorcluster, "socket out"=w295:refnum<class "zmq_socket.lvclass">, "context out"=w299:refnum<class "zmq_context.lvclass">)  [unwired: 2 in]
            n99 = Bundle By Name(cluster=w294, "ZMQ Context"=w299, "ZMQ Socket"=w295) -> (w300:T8)
            n100 = call <vilib>:"Add State(s) to Queue__jki_lib_state_machine.vi"("State(s) in (\"\")"=w305) -> ("States Out"=w304:string)  [unwired: 14 in]
          }
          frame "ZMQ: Create Socket" {
            # "This state is not \"create socket\";\nshould be named \"configure socket\""
            n101 = Unbundle By Name(w314) -> ("ZMQ Socket"=w311:refnum<class "zmq_socket.lvclass">, "Socket Config.Socket type"=w313:T6, "Socket Config.endpoint"=w312:string, "Socket Config.socket filter"=w307:string)
            n102 = case shown="\"ZMQ_SUB\"" w313 {
              tunnel: w312 -> [w324 w330 w338 w346 _]
              tunnel: w311 -> [w323 w334 w340 w345 w349]
              tunnel: w310 -> [w322 w332 w339 w344 w347]
              tunnel: [w320 w331 w335 w342 w347] -> w309
              tunnel: [w319 w333 w336 w341 w349] -> w308
              tunnel: w307 -> [_ w326 _ _ _]
              tunnel: [-1 ("T_O") 100 ("T_O") 100 ("T_O") 100 ("T_O") 0 ("T_O")] -> w306
              frame "ZMQ_PUB" {
                n103 = call <vilib>:"zmq_bind.vi"("error in"=w322, "endpoint"=w324, "socket in"=w323) -> ("error out"=w320:errorcluster, "socket out"=w319:refnum<class "zmq_socket.lvclass">)  [unwired: 1 in]
              }
              frame "ZMQ_SUB" {
                # "Consider\nexposing this\nto the user \nof the class"
                n104 = call <vilib>:"zmq_connect.vi"("error in"=w332, "endpoint"=w330, "socket in"=w334) -> ("error out"=w328:errorcluster, "socket out"=w327:refnum<class "zmq_socket.lvclass">)  [unwired: 1 in]
                n105 = call <vilib>:"zmq_setsocketopt.vi"("error in"=w328, "value"=w326, "option"=socket_options."ZMQ_SUBSCRIBE", "socket in"=w327) -> ("error out"=w331:errorcluster, "socket out"=w333:refnum<class "zmq_socket.lvclass">)  [unwired: 2 in]
              }
              frame "ZMQ_REQ" {
                # "Consider\nexposing this\nto the user \nof the class"
                n106 = call <vilib>:"zmq_connect.vi"("error in"=w339, "endpoint"=w338, "socket in"=w340) -> ("error out"=w335:errorcluster, "socket out"=w336:refnum<class "zmq_socket.lvclass">)  [unwired: 1 in]
              }
              frame "ZMQ_REP" {
                n107 = call <vilib>:"zmq_bind.vi"("error in"=w344, "endpoint"=w346, "socket in"=w345) -> ("error out"=w342:errorcluster, "socket out"=w341:refnum<class "zmq_socket.lvclass">)  [unwired: 1 in]
              }
              frame Default {
              }
            }
            n108 = Bundle By Name(cluster=w314, "ZMQ Socket"=w308, "T_O"=w306) -> (w315:T8)
            n109 = call <vilib>:"Add State(s) to Queue__jki_lib_state_machine.vi"("State(s) in (\"\")"=w318) -> ("States Out"=w317:string)  [unwired: 14 in]
          }
          frame "ZMQ: Close" {
            n110 = Unbundle By Name(w354) -> ("ZMQ Context"=w350:refnum<class "zmq_context.lvclass">, "ZMQ Socket"=w353:refnum<class "zmq_socket.lvclass">)
            n111 = call <vilib>:"zmq_close.vi"("error in"=w352, "socket"=w353) -> ("error out"=w355:errorcluster)  [unwired: 3 in]
            n112 = call <vilib>:"zmq_ctx_destroy.vi"("error in"=w355, "context in"=w350) -> ("error out"=w351:errorcluster)  [unwired: 3 in]
            n113 = call <vilib>:"Add State(s) to Queue__jki_lib_state_machine.vi"("State(s) in (\"\")"=w358) -> ("States Out"=w357:string)  [unwired: 14 in]
          }
          frame "ZMQ: Write" {
            # "Check if Write is valid"
            n114 = Unbundle By Name(w364) -> ("ZMQ Socket"=w363:refnum<class "zmq_socket.lvclass">, "Send String"=w360:string, "Socket Config.Socket type"=w359:T6)
            n115 = case shown="\"ZMQ_PUB\", \"ZMQ_REQ\", \"ZMQ_REP\"" w359 {
              tunnel: w363 -> [_ w372]
              tunnel: w362 -> [w368 w371]
              tunnel: [w368 w370] -> w361
              tunnel: w360 -> [_ w369]
              frame Default {
              }
              frame "ZMQ_PUB", "ZMQ_REQ", "ZMQ_REP" {
                n116 = call <vilib>:"zmq_send.vi"("error in"=w371, "data"=w369, "socket in"=w372) -> ("error out"=w370:errorcluster)  [unwired: 4 in, 1 out]
              }
            }
            n117 = call <vilib>:"Add State(s) to Queue__jki_lib_state_machine.vi"("State(s) in (\"\")"=w367) -> ("States Out"=w366:string)  [unwired: 14 in]
          }
          frame "ZMQ: Poll Sockets" {
            n118 = Unbundle By Name(w381) -> ("ZMQ Socket"=w377:refnum<class "zmq_socket.lvclass">, "Socket Config.Socket type"=w378:T6, "T_O"=w375:i32, "Self Reference"=w374:refnum<class "0MQ_Server.lvclass">)
            n119 = Unbundle By Name(w374) -> ("Incoming Message"=w373:refnum<user-event>)
            n120 = Build Array(w377) -> (w376:refnum<class "zmq_socket.lvclass">[])
            n121 = case shown="\"ZMQ_SUB\"..\"ZMQ_REP\"" w378 {
              tunnel: w376 -> [_ w388]
              tunnel: w380 -> [w385 w390]
              tunnel: [w385 w389] -> w379
              tunnel: w375 -> [_ w387]
              tunnel: w373 -> [_ w386]
              frame Default {
              }
              frame "ZMQ_SUB".."ZMQ_REP" {
                n122 = call <vilib>:"zmq_recv_event.vi"("error in"=w390, "timeout (none)"=w387, "sockets"=w388, "poll event"=w386) -> ("error out"=w389:errorcluster)  [unwired: 2 in, 1 out]
              }
            }
            n123 = call <vilib>:"Add State(s) to Queue__jki_lib_state_machine.vi"("State(s) in (\"\")"=w384) -> ("States Out"=w383:string)  [unwired: 14 in]
          }
        }
      }
    }
    frame Error {
    }
  }
  n124 = call-parent "Process.vi"("error in"=w7, "SMO"=w6) -> ("error out"=w4:errorcluster, "SMO out"=→"0MQ_Server out":refnum<class "0MQ_Server.lvclass">)  [unwired: 8 in]
  n125 = Merge Errors(w4, w3) -> (→"error out":errorcluster)
